vi "Configure Write Command RP Timeout.vi"(10 "Response Configuration in":T1) -> (2 "Response Configuration out":T1)   [LabVIEW 2017, in "SSH.lvlib"]
doc: "Allows the user to set a timeout longer than the default 5 seconds if needed."
uses:
  SSH.lvlib
  Response Configuration.ctl
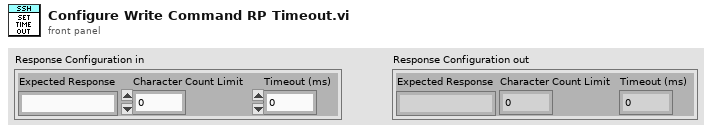
[diagram p1: front panel]
types:
  T1 = typedef "SSH.lvlib/Response Configuration.ctl" = cluster{"Expected Response":string, "Character Count Limit":i32, "Timeout (ms)":u32}
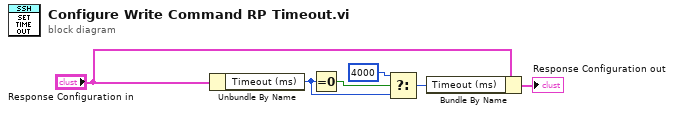
[diagram p0: block diagram]
diagram:
  n1 = Unbundle By Name("Response Configuration in") -> ("Timeout (ms)"=w5:u32)
  n2 = Equal To 0?(x=w5) -> (x = 0?=w6:bool)
  n3 = Select(t=u32 4000, s=w6, f=w5) -> (s? t:f=w2:u32)
  n4 = Bundle By Name(cluster="Response Configuration in", "Timeout (ms)"=w2) -> (→"Response Configuration out":T1)
